vi "Is Complete.vi"(8 "error in (no error)":errorcluster, 11 "Measure Controller in":refnum<class "Process Controller.lvclass">) -> (0 "error out":errorcluster, 3 "Measure Controller out":refnum<class "Process Controller.lvclass">)   [LabVIEW 2016, in "Process Controller.lvclass"]
uses:
  Process Controller.lvclass
  C:/github/Measure_core/Template Module/Template Module.lvclass
  C:/github/Measure_core/Worker/Worker.lvclass
  Process Controller.lvclass/Process Controller.ctl
  Template Module/Template Module.lvclass/Template Module.ctl
  Worker/Worker.lvclass/Worker.ctl
  Template Module/Read Reply to.vi
  Read Repeat times.vi
  Template Module/Read Active.vi
  Worker/Write Cycle count.vi
  Template Module Messages/Result Reply Msg/Result Reply Msg.lvclass
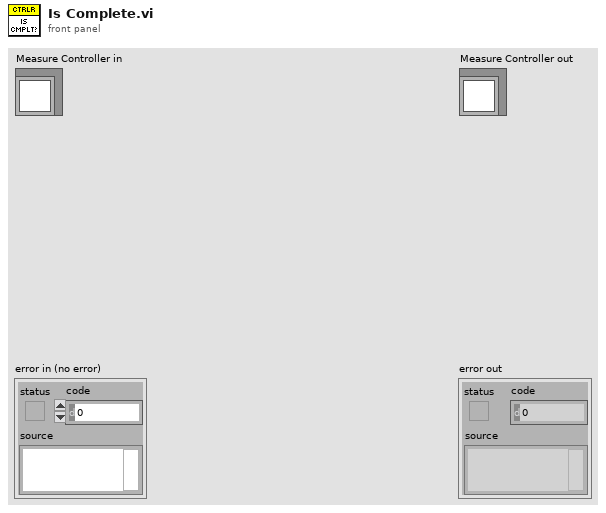
[diagram p1: front panel]
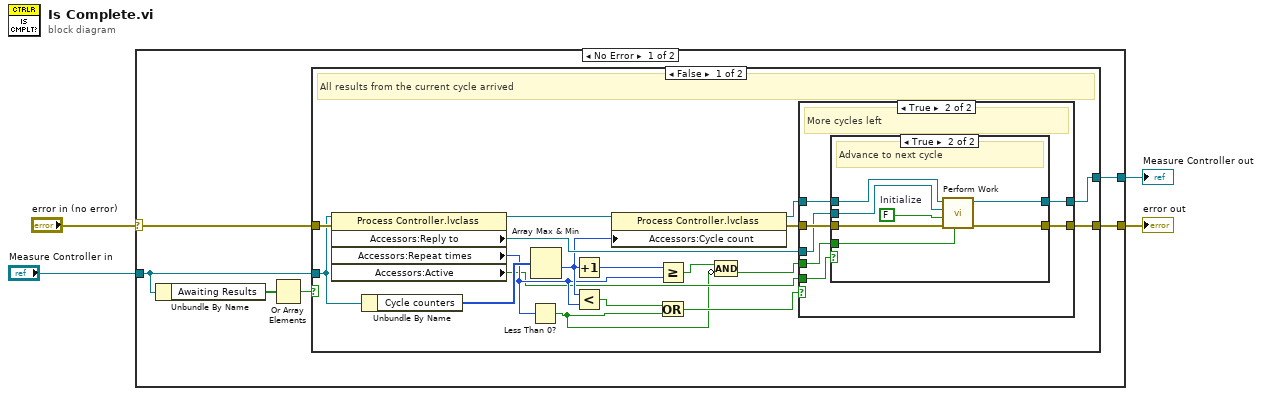
[diagram p0: block diagram]
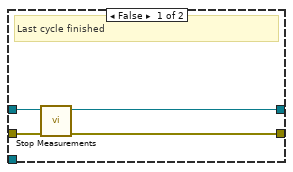
[diagram p2: hidden frame]
diagram:
  n1 = case shown="No Error" "error in (no error)" {
    selector: "error in (no error)" -> [w7 w52]
    tunnel: [w6 w52] -> w3
    tunnel: [w5 w51] -> w1
    tunnel: "Measure Controller in" -> [w8 w51]
    frame No Error {
      n2 = Unbundle By Name(w8) -> ("Awaiting Results"=w10:bool[])
      n3 = Or Array Elements(Boolean array=w10) -> (logical OR=w9:bool)
      n4 = case shown="False" w9 {
        tunnel: w8 -> [w18 w49]
        tunnel: w7 -> [w28 w50]
        tunnel: [w22 w50] -> w6
        tunnel: [w21 w49] -> w5
        frame False {
          # "All results from the current cycle arrived"
          n5 = property class="Process Controller.lvclass"(reference=w18, error in=w28) -> (reference out=w27:refnum<class "Process Controller.lvclass">, "Accessors:Reply to"=w20:refnum<class "Result Reply Msg.lvclass">, "Accessors:Repeat times"=w15:i32, "Accessors:Active"=w14:bool)  [unwired: 1 out]
          n6 = Unbundle By Name(w18) -> ("Cycle counters"=w17:i32[])
          n7 = Less Than 0?(x=w15) -> (x < 0?=w11:bool)
          n8 = Array Max & Min(array=w17) -> (min value=w16:i32)  [unwired: 3 out]
          n9 = Increment(x=w16) -> (x+1=w19:i32)
          n10 = Less?(x=w16, y=w15) -> (x < y?=w26:bool)
          n11 = property class="Process Controller.lvclass"(reference=w27, "Accessors:Cycle count"=w16) -> (reference out=w25:refnum<class "Process Controller.lvclass">, error out=w24:errorcluster)  [unwired: 1 in]
          n12 = Greater Or Equal?(x=w19, y=w15) -> (x >= y?=w12:bool)
          n13 = Or(x=w26, y=w11) -> (x .or. y?=w23:bool)
          n14 = Compound Arithmetic op=AND(w12, invert w11) -> (w13:bool)
          n15 = case shown="True" w23 {
            tunnel: w25 -> [w29 w39]
            tunnel: w24 -> [w32 w38]
            tunnel: [w31 w37] -> w22
            tunnel: [w30 w36] -> w21
            tunnel: w20 -> [_ w35]
            tunnel: w13 -> [_ w34]
            tunnel: w14 -> [_ w33]
            frame False {
              # "Last cycle finished"
              n16 = call-dynamic "Stop Measurements.vi"("error in (no error)"=w32, "Measure Controller in"=w29) -> ("error out"=w31:errorcluster, "Measure Controller out"=w30:refnum<class "Process Controller.lvclass">)  [unwired: 8 in]
            }
            frame True {
              # "More cycles left"
              n17 = case shown="True" w33 {
                tunnel: w39 -> [w40 w48]
                tunnel: w38 -> [w41 w47]
                tunnel: [w41 w46] -> w37
                tunnel: [w40 w45] -> w36
                tunnel: w35 -> [_ w43]
                tunnel: w34 -> [_ w42]
                frame False {
                  # "We are not active, do nothing"
                }
                frame True {
                  w44 = FALSE  # Initialize
                  # "Advance to next cycle"
                  n18 = call-dynamic "Perform Work.vi"("Last request"=w42, "error in (no error)"=w47, "Initialize"=w44, "Reply to"=w43, "Measure Controller in"=w48) -> ("error out"=w46:errorcluster, "Measure Controller out"=w45:refnum<class "Process Controller.lvclass">)  [unwired: 5 in]
                }
              }
            }
          }
        }
        frame True {
          # "Not all results from the current cycle arrived"
        }
      }
    }
    frame Error {
    }
  }
  "error out" <- w3
  "Measure Controller out" <- w1
